vi "Actor Core.vi"(8 "error in":errorcluster, 11 "TRExperimentsRaw in":refnum<class "TRExperimentsRaw.lvclass">) -> (0 "error out":errorcluster, 3 "Actor out":refnum<class "Actor.lvclass">)   [LabVIEW 2020, in "Forms.lvlib" / "TRExperimentsRaw.lvclass"]
doc: "The user interface for this panel.\n\n----\nPlease see the following web address for additional documentation and tutorial information:\nhttp://www.mooregoodideas.com/mgi-panel-manager/\n\nAuthor: Derek Trepanier\n\nCopyright (c) 2018, Moore Good Ideas, Inc.\n\nAll rights reserved.\n\nRedistribution and use in source and binary forms, with or without modification, are permitted provided that the following conditions are met:\n\n * Redistributions of source code must retain the above copyright notice, this list of conditions and the following disclaimer.\n * Redistributions in binary form must reproduce the above copyright notice, this list of conditions and the following disclaimer in the documentation and/or other materials provided with the distribution.\n * Neither the name of Moore Good Ideas, Inc. nor the names of its contributors may be used to endorse or promote products derived from this software without specific prior written permission.\n\nTHIS SOFTWARE IS PROVIDED BY THE COPYRIGHT HOLDERS AND CONTRIBUTORS \"AS IS\" AND ANY EXPRESS OR IMPLIED WARRANTIES, INCLUDING, BUT NOT LIMITED TO, THE IMPLIED WARRANTIES OF MERCHANTABILITY AND FITNESS FOR A PARTICULAR PURPOSE ARE DISCLAIMED. IN NO EVENT SHALL THE COPYRIGHT OWNER OR CONTRIBUTORS BE LIABLE FOR ANY DIRECT, INDIRECT, INCIDENTAL, SPECIAL, EXEMPLARY, OR CONSEQUENTIAL DAMAGES (INCLUDING, BUT NOT LIMITED TO, PROCUREMENT OF SUBSTITUTE GOODS OR SERVICES; LOSS OF USE, DATA, OR PROFITS; OR BUSINESS INTERRUPTION) HOWEVER CAUSED AND ON ANY THEORY OF LIABILITY, WHETHER IN CONTRACT, STRICT LIABILITY, OR TORT (INCLUDING NEGLIGENCE OR OTHERWISE) ARISING IN ANY WAY OUT OF THE USE OF THIS SOFTWARE, EVEN IF ADVISED OF THE POSSIBILITY OF SUCH DAMAGE."
uses:
  TRExperimentsRaw.lvclass
  C:/Users/User/Desktop/Raman Program/Database OOP/source/Forms AF/Forms Controller/Form Controller/Panel Form Controller.lvclass
  <vilib>/ActorFramework/Actor/Actor.lvclass
  Users/Users/Users.lvclass
  Samples/Samples.lvclass
  DataSets/DataSets Folder/DataSets.lvclass
  WorkingRange/Working Range.lvclass
  Forms Controller/Form Controller/Panel Form Controller.lvclass/Panel Form Controller.ctl
  Database OOP/Column Libraries/Basic Fields/Field Configurations/Field Configuration Class/Field Configuration.lvclass
  C:/Users/User/Desktop/Raman Program/Database OOP/source/Database OOP/Column Libraries/Field Interfaces/Field Configuration Interface Class/Field Configuration.lvclass
  Forms Controller/Open Form Button/Open Form Button.lvclass
  C:/Users/User/Desktop/Raman Program/Database OOP/source/Database OOP/Button Libraries/Button Interface Class/Button Interface.lvclass
  Database OOP/Column Libraries/Basic Field Constructors/Text Field.vi
  Database OOP/Column Libraries/Basic Field Constructors/FK Ring Field.vi
  Forms Controller/Form Window/Form Window.lvclass
  Forms Controller/Form Controller/Panel Form Controller.lvclass
  Database OOP/Table Libraries/Basic Form/Basic Form.lvclass
  Database OOP/Column Libraries/Basic Field Constructors.lvlib
panel:
  in  "Add Working Range":bool
  in  "Add Sample":bool
  in  "Add Data Set":bool
  in  "Add User":bool
  in  "Working Range":u16(ring) items=["None"=1]
  in  "Description":string
  in  "Sample":u16(ring) items=["None"=1, "P"=2, "BSP"=3, "R"=4, "OC"=5, "undoped"=6, "A"=7, "S"=8]
  in  "Data Set":u16(ring) items=["Chopper Phase"=1, "Solvent GS Raman"=2, "Raman Chirp Test"=3, "STO GS Raman"=4, "Program Test"=5, "Front vs Back Refl"=6, "OC ES Raman"=7, "CC ES Raman"=8, "Interfacial Water Test"=9]
  in  "User":u16(ring) items=["None"=1, "Michael"=2, "Suryansh"=3, "Ilya"=4, "Hanna"=5, "Tanja"=6]
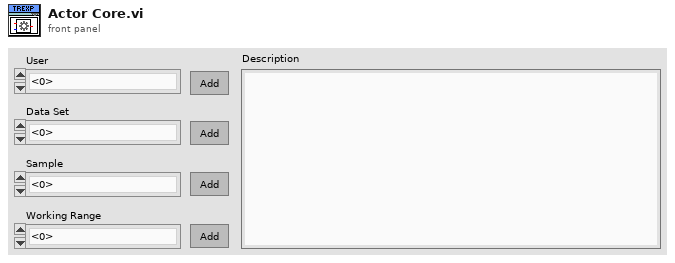
[diagram p1: front panel]
types:
  T1 = typedef "Panel Form Controller.lvlib/Builder Cluster.ctl" = cluster{"VI Ctrl Array":refnum<vi>[], "Form":refnum<class "Basic Form.lvclass">, "Open Form Button":refnum<class "Open Form Button.lvclass">}
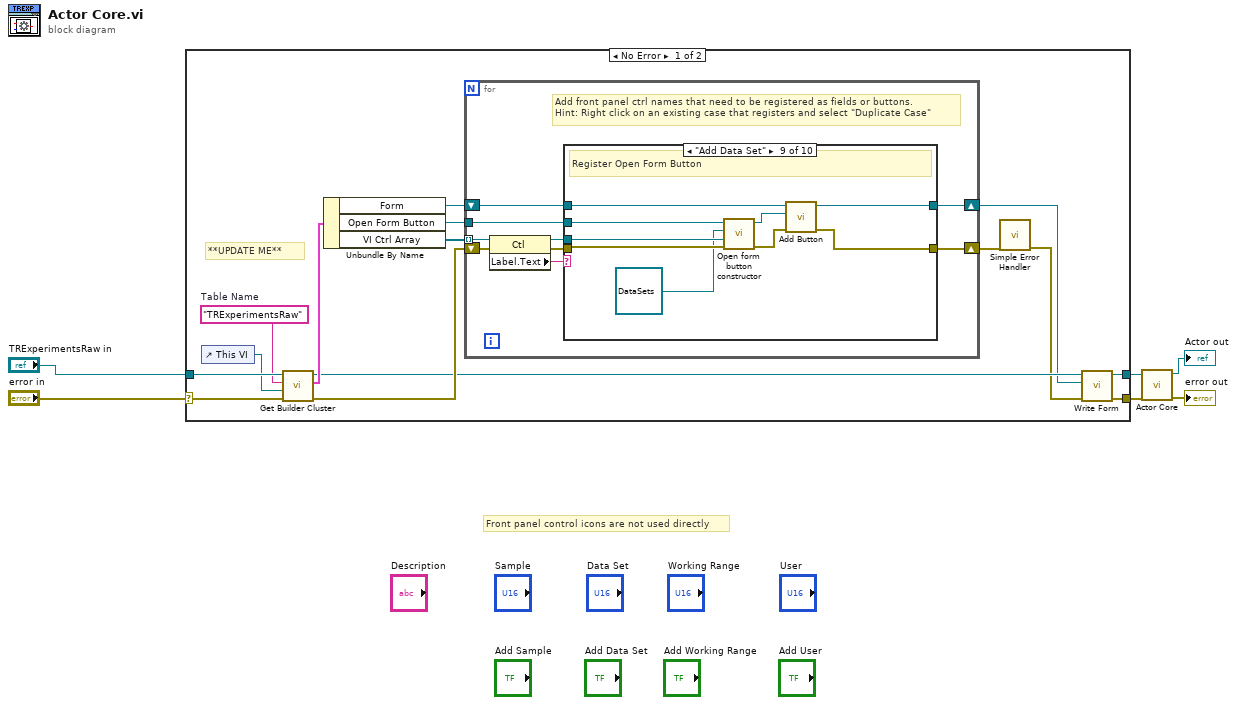
[diagram p0: block diagram]
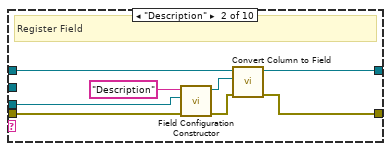
[diagram p3: hidden frame]
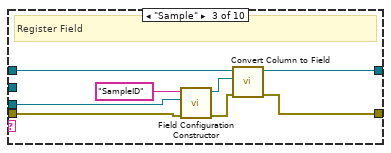
[diagram p4: hidden frame]
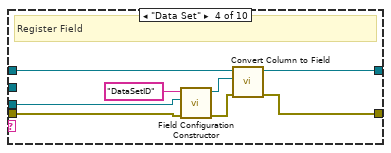
[diagram p5: hidden frame]
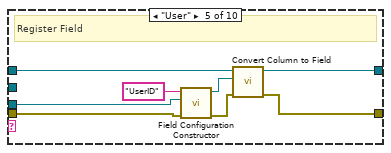
[diagram p6: hidden frame]
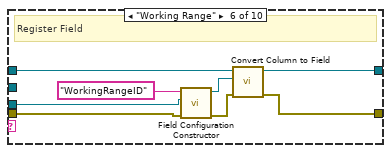
[diagram p7: hidden frame]
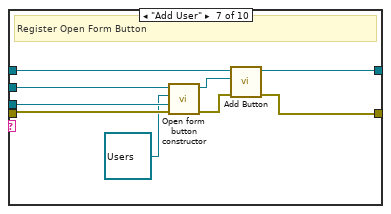
[diagram p8: hidden frame]
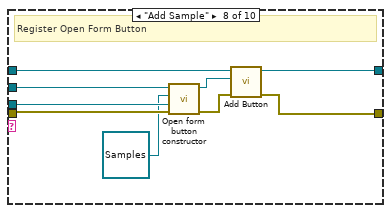
[diagram p9: hidden frame]
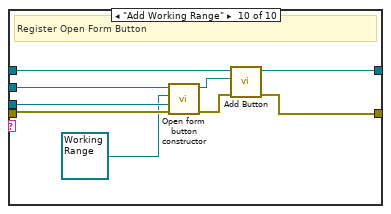
[diagram p10: hidden frame]
diagram:
  # "Front panel control icons are not used directly"
  n1 = case shown="No Error" "error in" {
    selector: "error in" -> [w17 w110]
    tunnel: "TRExperimentsRaw in" -> [w21 w109]
    tunnel: [w11 w110] -> w4
    tunnel: [w12 w109] -> w3
    frame No Error {
      w9 = "TRExperimentsRaw"  # Table Name
      # "**UPDATE ME**"
      n2 = control-ref of="This VI"() -> (w10:refnum<vi>)
      n3 = call "Get Builder Cluster.vi"("error in (no error)"=w17, "VI Refnum"=w10, "Table Name"=w9, "Panel Form Controller in"=w21) -> ("error out"=w19:errorcluster, "Builder Cluster"=w18:T1, "Panel Form Controller out"=w14:refnum<class "TRExperimentsRaw.lvclass">)  [unwired: 5 in]
      n4 = Unbundle By Name(w18) -> ("Form"=w20:refnum<class "Basic Form.lvclass">, "Open Form Button"=w15:refnum<class "Open Form Button.lvclass">, "VI Ctrl Array"=w16:refnum<vi>[])
      n5 = for {
        tunnel: w16 -> [w30] mode=indexing
        shift-right: [w24] -> w13
        shift-left: w20 -> [w25]
        shift-right: [w22] -> w8
        shift-left: w19 -> [w28]
        tunnel: w15 -> [w23]
        # "Add front panel ctrl names that need to be registered as fields or buttons.\nHint: Right click on an existing case that registers and select \"Duplicate Case\""
        n6 = property class="Ctl"(reference=w30, error in=w28) -> (reference out=w29:refnum<vi>, error out=w27:errorcluster, "Label.Text"=w26:string)
        n7 = case shown="\"Add Data Set\"" w26 {
          tunnel: w29 -> [_ w35 w44 w52 w60 w68 w75 w84 w93 w102]
          tunnel: w25 -> [w32 w40 w48 w56 w64 w72 w81 w90 w99 w108]
          tunnel: [w32 w38 w46 w54 w62 w70 w80 w89 w98 w107] -> w24
          tunnel: [w31 w39 w47 w55 w63 w71 w79 w88 w97 w106] -> w22
          tunnel: w27 -> [w31 w34 w43 w51 w59 w67 w74 w83 w92 w101]
          tunnel: w23 -> [_ _ _ _ _ _ w76 w85 w94 w103]
          frame "", Default {
            # "Not Registered"
          }
          frame "Description" {
            # "Register Field"
            n8 = call-poly "Field Configuration Constructor.vi"("error in"=w34, "Ctl Refnum"=w35, "Column Name"="Description" ("Column")) -> ("error out"=w37:errorcluster, "Field Configuration"=w33:refnum<class "Field Configuration.lvclass">)  [unwired: 7 in]
            n9 = call "Convert Column to Field.vi"("error in (no error)"=w37, "Field Configuration"=w33, "Basic Form in"=w40) -> ("error out"=w39:errorcluster, "Basic Form out"=w38:refnum<class "Basic Form.lvclass">)  [unwired: 7 in]
          }
          frame "Sample" {
            # "Register Field"
            n10 = call-poly "Field Configuration Constructor.vi"("error in"=w43, "Ctl Refnum"=w44, "Column Name"="SampleID" ("Column")) -> ("error out"=w45:errorcluster, "Field Configuration"=w42:refnum<class "Field Configuration.lvclass">)  [unwired: 7 in]
            n11 = call "Convert Column to Field.vi"("error in (no error)"=w45, "Field Configuration"=w42, "Basic Form in"=w48) -> ("error out"=w47:errorcluster, "Basic Form out"=w46:refnum<class "Basic Form.lvclass">)  [unwired: 7 in]
          }
          frame "Data Set" {
            # "Register Field"
            n12 = call-poly "Field Configuration Constructor.vi"("error in"=w51, "Ctl Refnum"=w52, "Column Name"="DataSetID" ("Column")) -> ("error out"=w53:errorcluster, "Field Configuration"=w50:refnum<class "Field Configuration.lvclass">)  [unwired: 7 in]
            n13 = call "Convert Column to Field.vi"("error in (no error)"=w53, "Field Configuration"=w50, "Basic Form in"=w56) -> ("error out"=w55:errorcluster, "Basic Form out"=w54:refnum<class "Basic Form.lvclass">)  [unwired: 7 in]
          }
          frame "User" {
            # "Register Field"
            n14 = call-poly "Field Configuration Constructor.vi"("error in"=w59, "Ctl Refnum"=w60, "Column Name"="UserID" ("Column")) -> ("error out"=w61:errorcluster, "Field Configuration"=w58:refnum<class "Field Configuration.lvclass">)  [unwired: 7 in]
            n15 = call "Convert Column to Field.vi"("error in (no error)"=w61, "Field Configuration"=w58, "Basic Form in"=w64) -> ("error out"=w63:errorcluster, "Basic Form out"=w62:refnum<class "Basic Form.lvclass">)  [unwired: 7 in]
          }
          frame "Working Range" {
            # "Register Field"
            n16 = call-poly "Field Configuration Constructor.vi"("error in"=w67, "Ctl Refnum"=w68, "Column Name"="WorkingRangeID" ("Column")) -> ("error out"=w69:errorcluster, "Field Configuration"=w66:refnum<class "Field Configuration.lvclass">)  [unwired: 7 in]
            n17 = call "Convert Column to Field.vi"("error in (no error)"=w69, "Field Configuration"=w66, "Basic Form in"=w72) -> ("error out"=w71:errorcluster, "Basic Form out"=w70:refnum<class "Basic Form.lvclass">)  [unwired: 7 in]
          }
          frame "Add User" {
            # "Register Open Form Button"
            n18 = call "Open form button constructor.vi"("error in (no error)"=w74, "Ctl Refnum"=w75, "Panel Form"=refnum<class "Users.lvclass"> refnum ("Forms.lvlib:Users.lvclass"), "Open Form Button in"=w76) -> ("error out"=w77:errorcluster, "Open Form Button out"=w78:refnum<class "Open Form Button.lvclass">)  [unwired: 6 in]
            n19 = call "Add Button.vi"("error in (no error)"=w77, "Button"=w78, "Basic Form in"=w81) -> ("error out"=w79:errorcluster, "Basic Form out"=w80:refnum<class "Basic Form.lvclass">)  [unwired: 7 in]
          }
          frame "Add Sample" {
            # "Register Open Form Button"
            n20 = call "Open form button constructor.vi"("error in (no error)"=w83, "Ctl Refnum"=w84, "Panel Form"=refnum<class "Samples.lvclass"> refnum ("Forms.lvlib:Samples.lvclass"), "Open Form Button in"=w85) -> ("error out"=w86:errorcluster, "Open Form Button out"=w87:refnum<class "Open Form Button.lvclass">)  [unwired: 6 in]
            n21 = call "Add Button.vi"("error in (no error)"=w86, "Button"=w87, "Basic Form in"=w90) -> ("error out"=w88:errorcluster, "Basic Form out"=w89:refnum<class "Basic Form.lvclass">)  [unwired: 7 in]
          }
          frame "Add Data Set" {
            # "Register Open Form Button"
            n22 = call "Open form button constructor.vi"("error in (no error)"=w92, "Ctl Refnum"=w93, "Panel Form"=refnum<class "DataSets.lvclass"> refnum ("Forms.lvlib:DataSets.lvclass"), "Open Form Button in"=w94) -> ("error out"=w95:errorcluster, "Open Form Button out"=w96:refnum<class "Open Form Button.lvclass">)  [unwired: 6 in]
            n23 = call "Add Button.vi"("error in (no error)"=w95, "Button"=w96, "Basic Form in"=w99) -> ("error out"=w97:errorcluster, "Basic Form out"=w98:refnum<class "Basic Form.lvclass">)  [unwired: 7 in]
          }
          frame "Add Working Range" {
            # "Register Open Form Button"
            n24 = call "Open form button constructor.vi"("error in (no error)"=w101, "Ctl Refnum"=w102, "Panel Form"=refnum<class "Working Range.lvclass"> refnum ("Forms.lvlib:Working Range.lvclass"), "Open Form Button in"=w103) -> ("error out"=w104:errorcluster, "Open Form Button out"=w105:refnum<class "Open Form Button.lvclass">)  [unwired: 6 in]
            n25 = call "Add Button.vi"("error in (no error)"=w104, "Button"=w105, "Basic Form in"=w108) -> ("error out"=w106:errorcluster, "Basic Form out"=w107:refnum<class "Basic Form.lvclass">)  [unwired: 7 in]
          }
        }
      }
      n26 = call <vilib>:"Simple Error Handler.vi"("error in (no error)"=w8) -> ("error out"=w7:errorcluster)  [unwired: 4 in, 4 out]
      n27 = call "Write Form.vi"("error in (no error)"=w7, "Form.lvlib:Basic Form.lvclass"=w13, "Panel Form Controller in"=w14) -> ("error out"=w11:errorcluster, "Panel Form Controller out"=w12:refnum<class "TRExperimentsRaw.lvclass">)  [unwired: 7 in]
    }
    frame Error {
    }
  }
  n28 = call-parent "Actor Core.vi"("error in"=w4, "Form Window in"=w3) -> ("error out"=→"error out":errorcluster, "Actor out"=→"Actor out":refnum<class "Actor.lvclass">)  [unwired: 8 in]
